vi "Init_Save.vi"(8 "Error In":errorcluster) -> (0 "Error Out":errorcluster, 3 "Queue Cluster":T1)   [LabVIEW 2021, in "Queues.lvlib"]
doc: "This subVI is used to init the queue and user event of the Save VI"
uses:
  Queues.lvlib
  Tipski Definicii/Save_program_queues.ctl
  Tipski Definicii/Save_Sostojbi.ctl
panel:
  # "Output"
  # "Input"
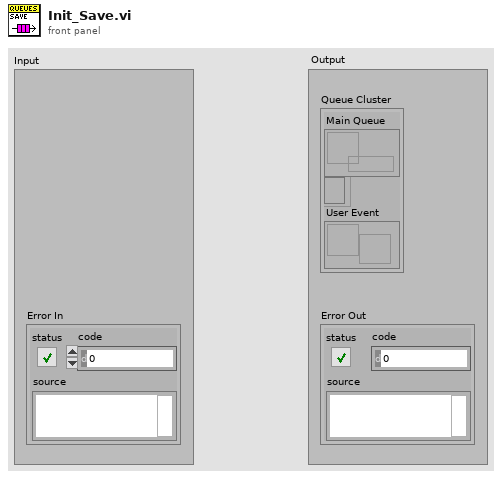
[diagram p1: front panel]
types:
  T1 = typedef "Save_program_queues.ctl" = cluster{"Main Queue":refnum<queue>, "ER Refnum":refnum<event-registration>, "User Event":refnum<user-event>}
  T2 = typedef "Save_Sostojbi.ctl" = enum16{"Init", "Generate Message", "Pick Path", "Save", "End"}
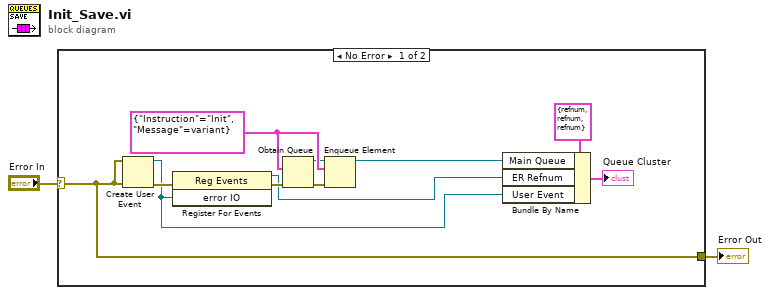
[diagram p0: block diagram]
diagram:
  n1 = case shown="No Error" "Error In" {
    selector: "Error In" -> [w3 w14]
    tunnel: [w3 w14] -> w1
    frame No Error {
      w11 = cluster{"Instruction":T2, "Message":variant} {"Instruction"=enum."Init", "Message"=variant}
      n2 = Create User Event(user event datatype=w3, error in=w3) -> (user event=w5:refnum<user-event>, error out=w12:errorcluster)
      n3 = register-events(error in=w12, w5) -> (reference out=w6:refnum<event-registration>, error out=w13:errorcluster)  [unwired: 1 in]
      n4 = Obtain Queue(element data type=w11, error in (no error)=w13) -> (queue out=w10:refnum<queue>, error out=w9:errorcluster)  [unwired: 3 in, 1 out]
      n5 = Enqueue Element(queue=w10, element=w11, error in (no error)=w9) -> (queue out=w7:refnum<queue>)  [unwired: 1 in, 2 out]
      n6 = Bundle By Name(cluster=T1 {"Main Queue"=refnum, "ER Refnum"=refnum, "User Event"=refnum}, "Main Queue"=w7, "ER Refnum"=w6, "User Event"=w5) -> (→"Queue Cluster":T1)
    }
    frame Error {
    }
  }
  "Error Out" <- w1
